vi "DSF.Engine.Framework.Initialize Inline Buffer.vi"(8 "error in (no error)":errorcluster, 9 "channel count":u64, 10 "first channel offset":u64, 11 "Framework in":refnum<class "VeriStand Framework.lvclass">) -> (0 "error out":errorcluster, 2 "Buffer":refnum<class "DSF.Engine.Pointer.DBL.lvclass">, 3 "Framework out":refnum<class "VeriStand Framework.lvclass">)   [LabVIEW 2017, in "Data Sharing Framework Engine.lvlib" / "VeriStand Framework.lvclass"]
uses:
  VeriStand Framework.lvclass
  dsf core/Built/DSF.Engine.lvlibp/Engine/Classes/Pointer/DSF.Engine.Pointer.DBL.lvclass
  dsf core/Built/DSF.Engine.lvlibp/Engine/Classes/Framework/DSF.Engine.Framework.lvclass
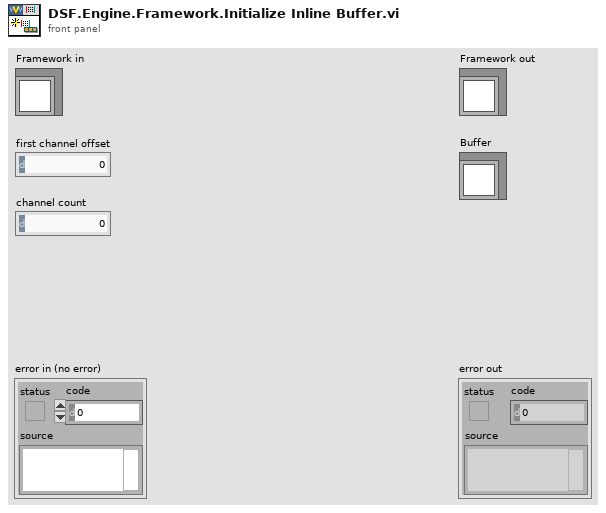
[diagram p1: front panel]
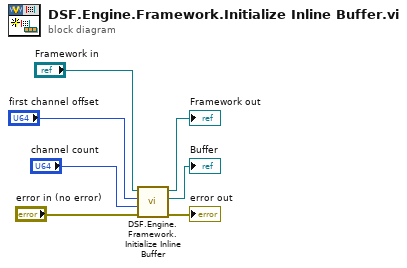
[diagram p0: block diagram]
diagram:
  n1 = call-parent "DSF.Engine.Framework.Initialize Inline Buffer.vi"("error in (no error)"="error in (no error)", "channel count"="channel count", "first channel offset"="first channel offset", "Framework in"="Framework in") -> ("error out"=→"error out":errorcluster, "Buffer"=→"Buffer":refnum<class "DSF.Engine.Pointer.DBL.lvclass">, "Framework out"=→"Framework out":refnum<class "VeriStand Framework.lvclass">)  [unwired: 5 in]
